vi "Test Update.vi"(8 "error in (no error)":errorcluster, 10 "Test Record":T2, 11 "Connection Refnum":T1) -> (0 "error out":errorcluster, 3 "Connection Refnum":T1)   [LabVIEW 2011]
uses:
  Test Record.ctl
  Summitek EXT/ODBC/SQL Controls/Connection Refnum.ctl
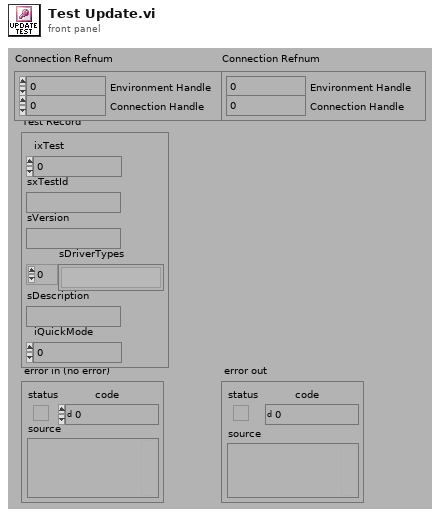
[diagram p1: front panel]
types:
  T1 = typedef "Connection Refnum.ctl" = cluster{"Environment Handle":i32, "Connection Handle":i32}
  T2 = typedef "Test Record.ctl" = cluster{"ixTest":i32, "sxTestId":string, "sVersion":string, "sDriverTypes":string[], "sDescription":string, "iQuickMode":i32}
  T3 = typedef "Statement Refnum.ctl" = cluster{"Statement Handle":i32, "Parameter Number":u16}
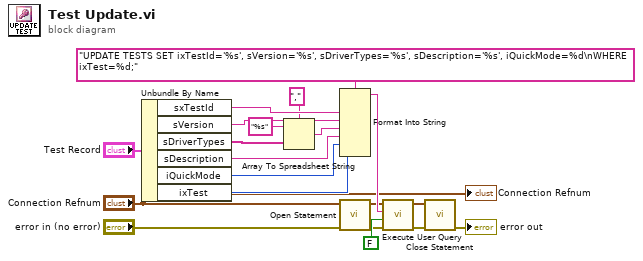
[diagram p0: block diagram]
diagram:
  n1 = Unbundle By Name("Test Record") -> ("sxTestId"=w14:string, "sVersion"=w13:string, "sDriverTypes"=w8:string[], "sDescription"=w9:string, "iQuickMode"=w4:i32, "ixTest"=w10:i32)
  n2 = Array To Spreadsheet String(delimiter (Tab)=",", array=w8, 3:"%s" ("format string")) -> (spreadsheet string=w5:string)
  n3 = Format Into String(format string="UPDATE TESTS SET ixTestId='%s', sVersion='%s', sDriverTypes='%s', sDescription='%s', iQuickMode=%d\nWHERE ixTest=%d;" ("User Query"), w14, w13, w5, w9, w4, w10) -> (resulting string=w15:string)  [unwired: 2 in, 1 out]
  n4 = call "Open Statement.vi"("error in (no error)"="error in (no error)", "Connection Refnum"="Connection Refnum") -> ("error out"=w12:errorcluster, "Statement Refnum"=w11:T3)  [unwired: 4 out]
  n5 = call "Execute User Query.vi"("error in (no error)"=w12, "Return Data? (f)"=FALSE, "User Query"=w15, "Statement Refnum"=w11) -> ("error out"=w18:errorcluster, "Statement Refnum"=w17:T3)  [unwired: 2 out]
  n6 = call "Close Statement.vi"("error in (no error)"=w18, "Statement Refnum"=w17) -> ("error out"=→"error out":errorcluster)  [unwired: 5 out]
  "Connection Refnum" <- "Connection Refnum"
